vi "new_P44.vi"(9 "new_offset":bool, 10 "P44":fxp<+,32,16>, 11 "E44":fxp<+,32,16>) -> (1 "output valid":bool, 3 "new_P44":fxp<+,32,16>)   [LabVIEW 2020]
uses:
  <vilib>/rvi/FXPMathLib/FxpAdd/XNode/nifxpmath_Add.xnode
  <vilib>/rvi/FXPMathLib/sim/FxpSim.dll
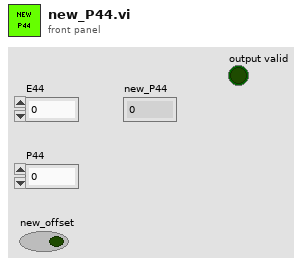
[diagram p1: front panel]
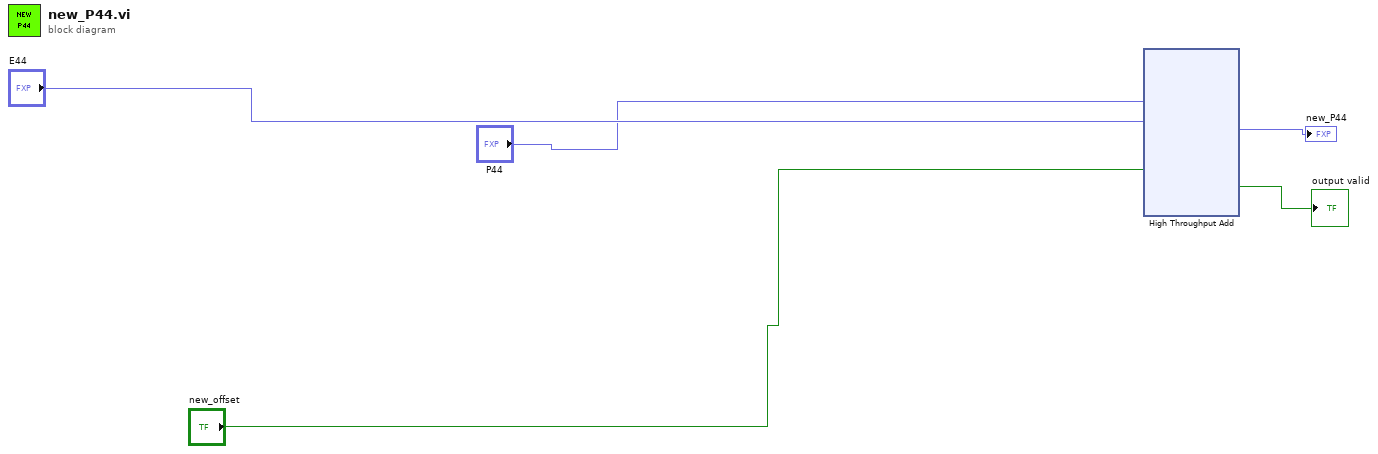
[diagram p0: block diagram]
diagram:
  n1 = xnode "High Throughput Add"("x"="P44", "y"="E44", "input valid"="new_offset") -> ("x+y"=→"new_P44":fxp<+,32,16>, "output valid"=→"output valid":bool)  [unwired: 1 in, 1 out]
